vi "U6 Multiple AIN Example.vi"() -> ()   [LabVIEW 2021]
panel:
  in  "Binary":bool
  in  "SettlingFactor":i32
  in  "Negative Channels":i32[](array[numeric])=[0, 0, 0, 0]
  in  "Ranges":string[](array[string])=["LJ_rgBIP10V", "LJ_rgBIP10V", "LJ_rgBIPP01V", "LJ_rgBIPP01V"]
  in  "Positive Channels":i32[](array[numeric])=[0, 1, 2, 3]
  out "Values Read":dbl[](array[numeric]) format="%.6f"
  out "Error Message":string
  in  "Resolution":i32
  out "error out":errorcluster
  # "Aquires multiple analog input channels over USB from the first found U6.\n\nThis uses the LabVIEW utility AddS-Go-Get.vi, rather than calling eAddGoGet from the UD driver.  The utility\nVI has better/easier error handling and is normally preferred, but eAddGoGet is a single call to the UD driver\nso often preferred if you will have parallel driver calls to the same handle within the same thread (none of\nour examples do this)."
  # "LJ_rgBIP10V\nLJ_rgBIP1V\nLJ_rgBIPP1V\nLJ_rgBIPP01V"
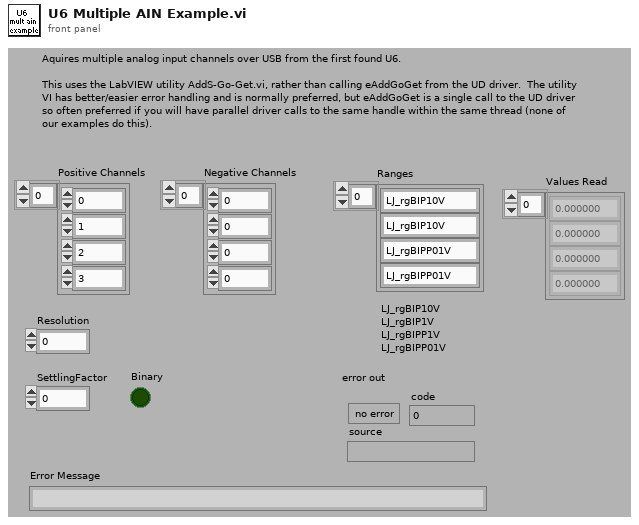
[diagram p1: front panel]
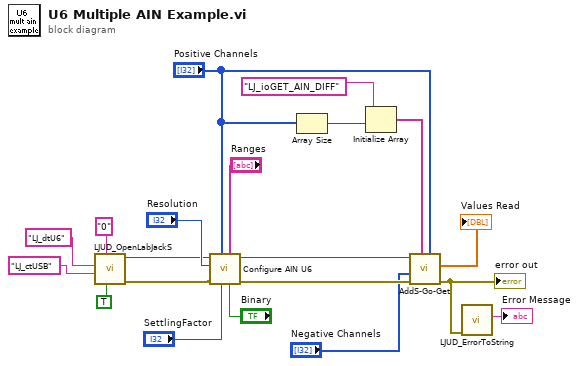
[diagram p0: block diagram]
diagram:
  n1 = call "LJUD_OpenLabJackS.vi"("FirstFound"=TRUE, "Address"="0", "ConnectionType"="LJ_ctUSB", "DeviceType"="LJ_dtU6") -> ("error out"=w8:errorcluster, "Handle"=w9:i32)  [unwired: 5 in, 1 out]
  n2 = call "Configure AIN U6.vi"("Binary"="Binary", "Ranges"="Ranges", "SettlingFactor"="SettlingFactor", "Positive Channels"="Positive Channels", "error in"=w8, "Resolution"="Resolution", "Handle In"=w9) -> ("error out"=w17:errorcluster, "Handle Out"=w18:i32)  [unwired: 3 in]
  n3 = Array Size(array="Positive Channels") -> (size(s)=w5:i32)
  n4 = Initialize Array("LJ_ioGET_AIN_DIFF" ("IOType"), w5) -> (w6:string[])
  n5 = call "AddS-Go-Get.vi"("Channels"="Positive Channels", "IOTypes"=w6, "error in"=w17, "x1"="Negative Channels", "Handle In"=w18) -> ("error out"=w16:errorcluster, "Values Read"=→"Values Read":dbl[])  [unwired: 4 in, 1 out]
  "error out" <- w16
  n6 = call "LJUD_ErrorToString.vi"("error in"=w16) -> ("String"=→"Error Message":string)  [unwired: 10 in]
